vi "Magnitude.vi"(11 "A":refnum<class "Vector 2D.lvclass">) -> (3 "Magnitude":sgl)   [LabVIEW 2021, in "Vector 2D.lvclass"]
uses:
  Vector 2D.lvclass
  Vector 2D.lvclass/Vector 2D.ctl
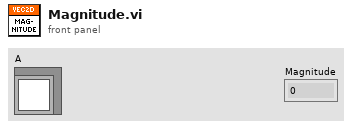
[diagram p1: front panel]
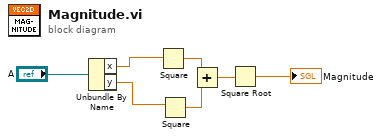
[diagram p0: block diagram]
diagram:
  n1 = Unbundle By Name("A") -> ("x"=w3:sgl, "y"=w2:sgl)
  n2 = Square(x=w3) -> (x^2=w5:sgl)
  n3 = Square(x=w2) -> (x^2=w6:sgl)
  n4 = Add(x=w5, y=w6) -> (x+y=w7:sgl)
  n5 = Square Root(x=w7) -> (sqrt(x)=→"Magnitude":sgl)
